vi "FY6900.vi"(4 "Error In":errorcluster, 7 "Command":T13) -> (0 "Error Out":errorcluster, 3 "Response":T11)   [LabVIEW 2018]
uses:
  MOKO_LabViewLibrary/MokoLowLevel/MokoLowLovelControl/MLLC_Command.ctl
  MOKO_LabViewLibrary/MokoLowLevel/MokoLowLovelControl/MLLC_Mode.ctl
  MOKO_LabViewLibrary/MokoLowLevel/MokoLowLovelControl/MLLC_Response.ctl
  MOKO_LabViewLibrary/MokoLowLevel/MokoLowLovelControl/MLLC_ConnectCluster.ctl
  MOKO_LabViewLibrary/MokoLowLevel/MokoLowLovelControl/MLLC_InterfaceType.ctl
  MOKO_LabViewLibrary/MokoLowLevel/MokoLowLovelControl/MLLC_OpenedSession.ctl
  MOKO_LabViewLibrary/MokoLowLevel/MokoLowLovelControl/MLLC_InterfaceSettings.ctl
  MOKO_LabViewLibrary/MokoLowLevel/MokoLowLovelControl/MLLC_InterfaceKind.ctl
  MOKO_LabViewLibrary/MokoLowLevel/MokoLowLovelControl/MLLC_DriverName.ctl
  MOKO_LabViewLibrary/MokoLowLevel/MokoLowLovelControl/MLLC_ResponseInit.ctl
  MOKO_LabViewLibrary/MokoLowLevel/MokoLowLovelControl/MLLC_Request.ctl
  MOKO_LabViewLibrary/MokoLowLevel/MokoLowLovelControl/MLLC_ErrorCode.ctl
  MOKO_LabViewLibrary/MokoLowLevel/MokoLowLovelControl/MLLC_Rs232Settings.ctl
panel:
  in  "Error Code":T1=5420
  in  "Request":T2="UMO"
  in  "ResponseInit":T3="FY6900"
  in  "Driver Name":T4="FY6900"
  in  "Settings":T10={"Saved Data"=variant, "Permanent data"={"Connect"={"InterfaceType"=enum."VISA", "OpenedSession"="", "InterfaceSettings"={"Interface"=enum."RS232", "EOS 4 read"=enum."LF (\\n)", "EOS 4 write"=enum."LF (\\n)", "TMO, ms"=2000, "Sett"=variant(cluster{"Baud Rate":u32, "Data Bits":u16, "Parity":u16, "Stop Bits":u16, "Flow Control":u16, "Eho":bool} {"Baud Rate"=75, "Data Bits"=0, "Parity"=0, "Stop Bits"=0, "Flow Control"=0, "Eho"=FALSE})}}}}
  in  "Mode":T12=enum."Check"
  # "FY6900"
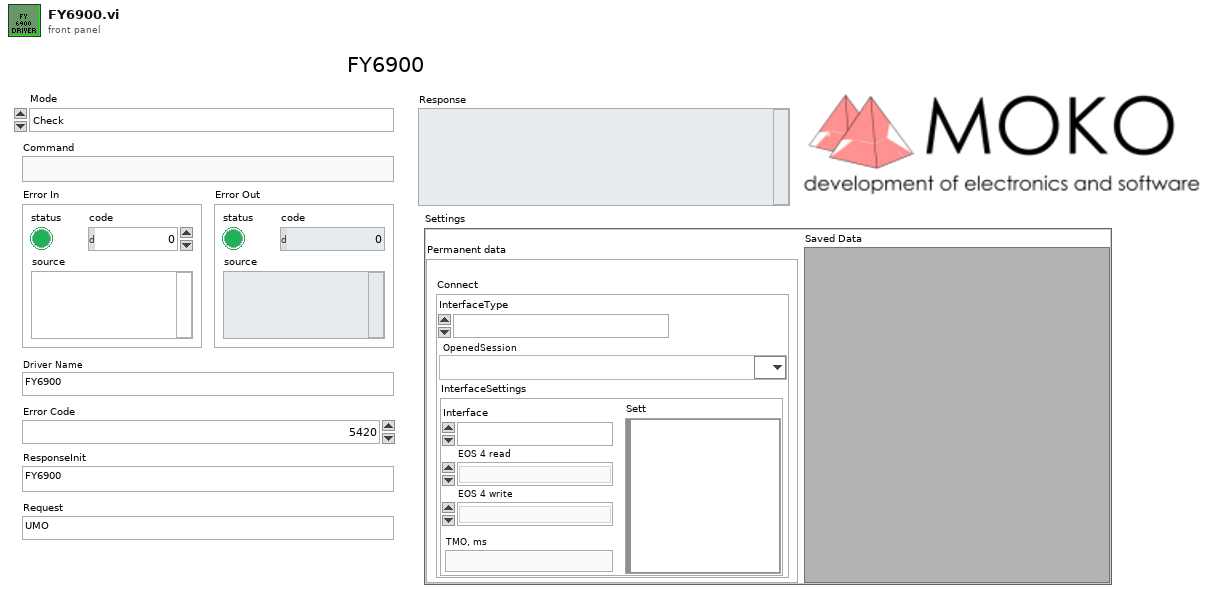
[diagram p1: front panel]
types:
  T1 = typedef "MLLC_ErrorCode.ctl" = u32
  T2 = typedef "MLLC_Request.ctl" = string
  T3 = typedef "MLLC_ResponseInit.ctl" = string
  T4 = typedef "MLLC_DriverName.ctl" = string
  T5 = typedef "MLLC_ConnectCluster.ctl" = cluster{"InterfaceType":T6, "OpenedSession":T7, "InterfaceSettings":T8}
  T6 = typedef "MLLC_InterfaceType.ctl" = enum16{"VISA", "Prologix USB-GPIB"}
  T7 = typedef "MLLC_OpenedSession.ctl" = refnum<visa-resource-name>
  T8 = typedef "MLLC_InterfaceSettings.ctl" = cluster{"Interface":T9, "EOS 4 read":enum16{"Default (=EOS 4 write)", "CR (\\r)", "LF (\\n)", "None"}, "EOS 4 write":enum16{"CR+LF (\\r\\n)", "CR (\\r)", "LF (\\n)", "None"}, "TMO, ms":i32, "Sett":variant}
  T9 = typedef "MLLC_InterfaceKind.ctl" = enum16{"RS232", "GPIB", "USB", "Ethernet", "another"}
  T10 = cluster{"Saved Data":variant, "Permanent data":cluster{"Connect":T5}}
  T11 = typedef "MLLC_Response.ctl" = string
  T12 = typedef "MLLC_Mode.ctl" = enum16{"get", "set", "close", "Init", "Check"}
  T13 = typedef "MLLC_Command.ctl" = string
  T14 = enum16{"CR+LF (\\r\\n)", "CR (\\r)", "LF (\\n)", "None"}
  T15 = enum16{"Default (=EOS 4 write)", "CR (\\r)", "LF (\\n)", "None"}
  T16 = typedef "MLLC_Error.ctl" = errorcluster
  T17 = typedef "MLLC_Rs232Settings.ctl" = cluster{"Baud Rate":u32, "Data Bits":u16, "Parity":u16, "Stop Bits":u16, "Flow Control":u16, "Eho":bool}
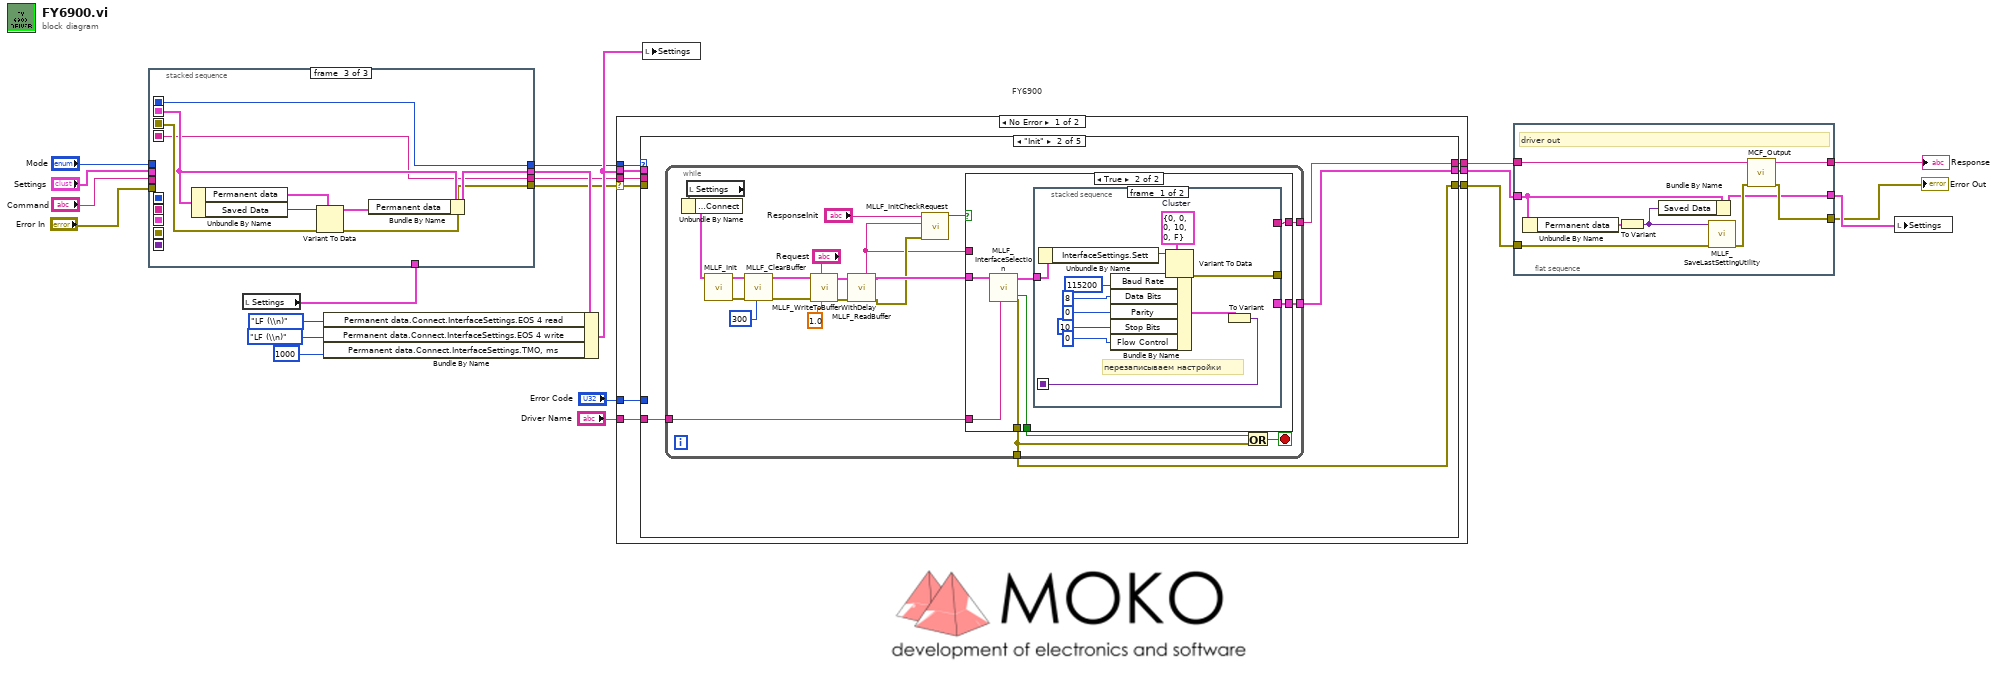
[diagram p0: block diagram]
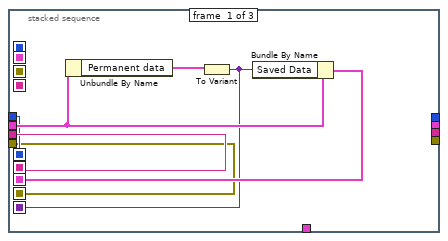
[diagram p2: hidden frame]
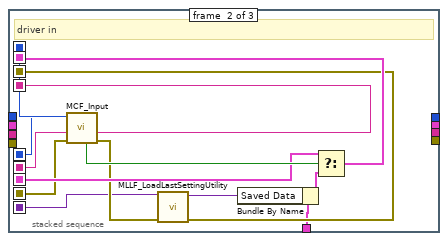
[diagram p3: hidden frame]
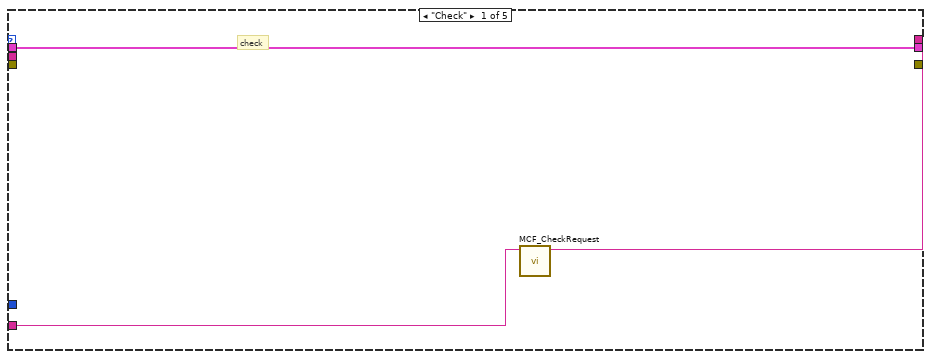
[diagram p4: hidden frame]
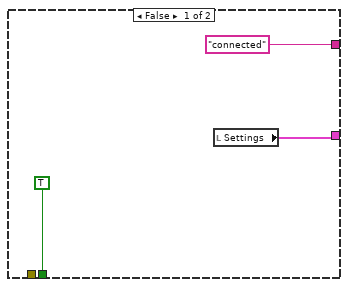
[diagram p5: hidden frame]
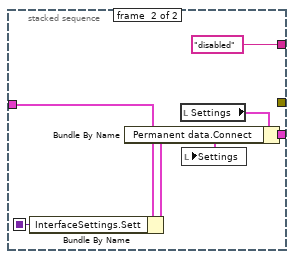
[diagram p6: hidden frame]
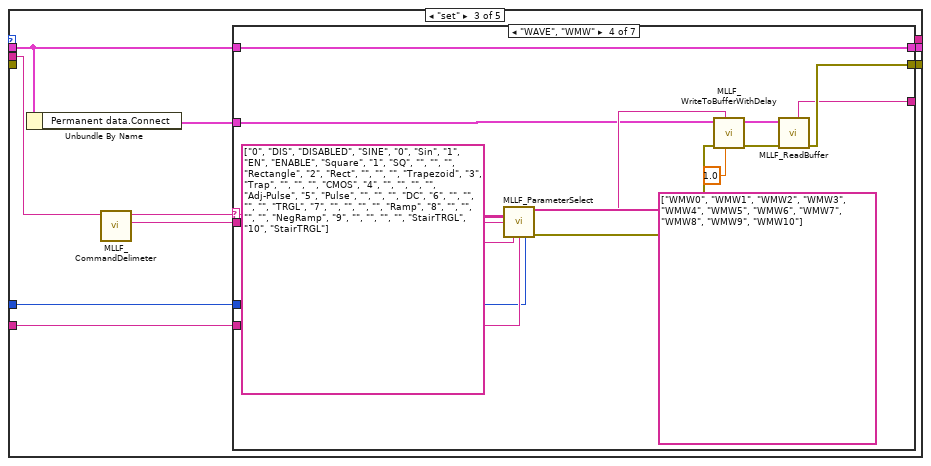
[diagram p7: hidden frame]
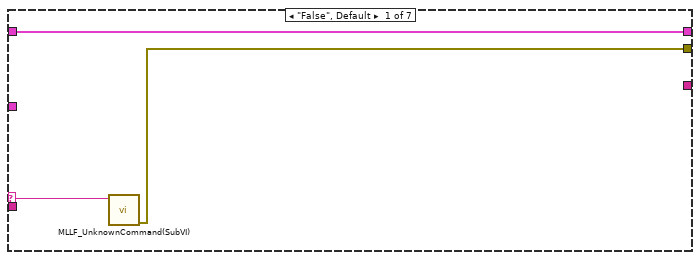
[diagram p8: hidden frame]
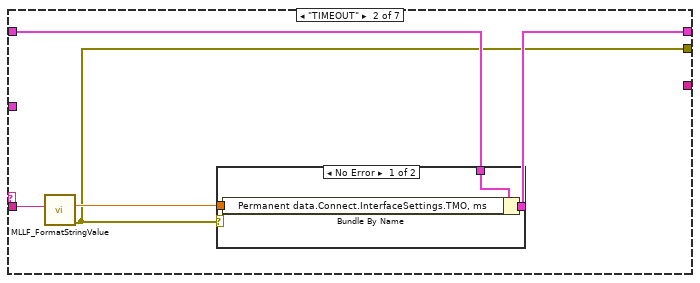
[diagram p9: hidden frame]
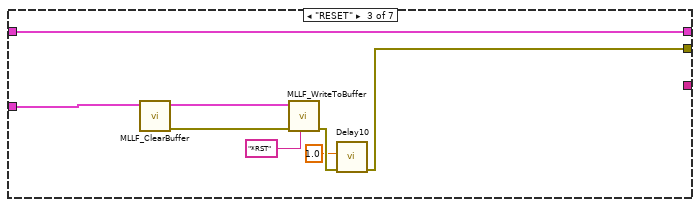
[diagram p11: hidden frame]
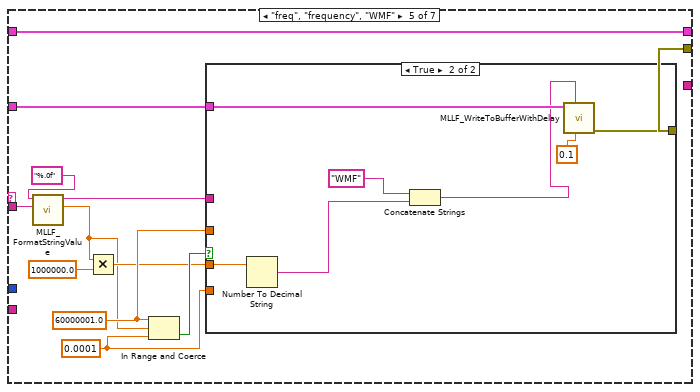
[diagram p12: hidden frame]
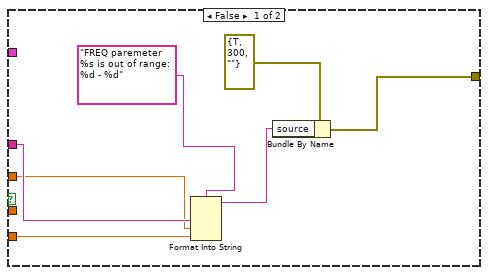
[diagram p13: hidden frame]
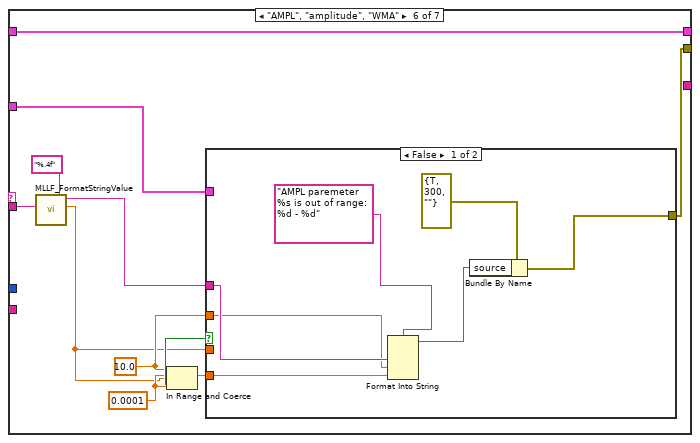
[diagram p14: hidden frame]
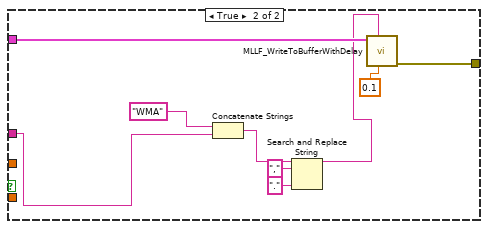
[diagram p15: hidden frame]
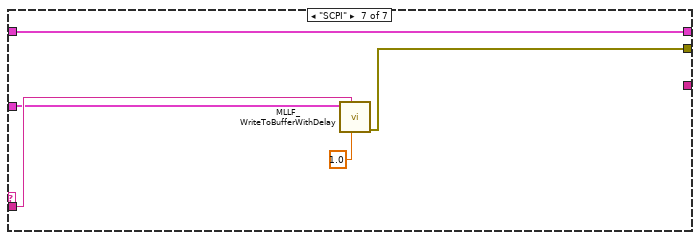
[diagram p16: hidden frame]
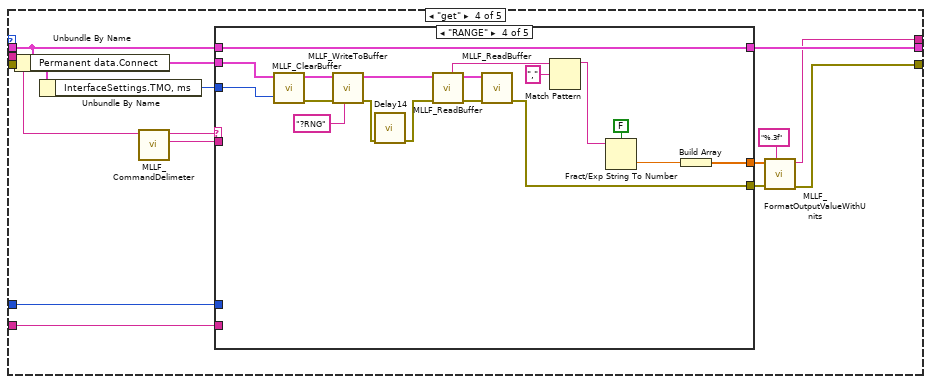
[diagram p17: hidden frame]
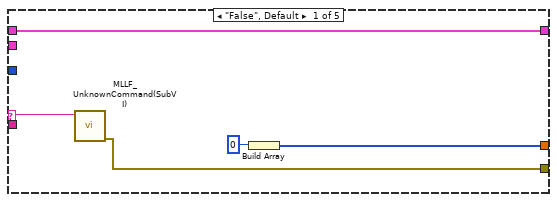
[diagram p18: hidden frame]
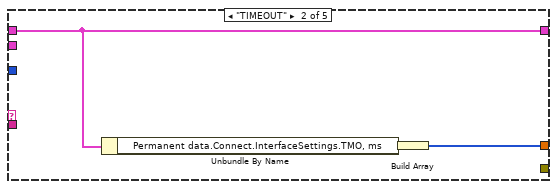
[diagram p19: hidden frame]
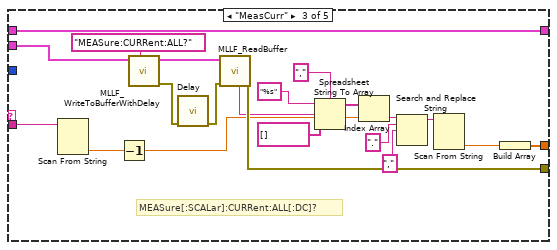
[diagram p20: hidden frame]
diagram:
  # "FY6900"
  n1 = local read "Settings"() -> (w5:T10)
  n2 = stacked-sequence {
    seq-local: [w24 _ _] -> [_ w40 _]
    seq-local: [w23 _ _] -> [_ w41 _]
    seq-local: [w26 _ _] -> [_ w36 _]
    seq-local: [w22 _ _] -> [_ w35 _]
    seq-local: [w25 _ _] -> [_ w31 _]
    seq-local: [_ w32 _] -> [_ _ w48]
    seq-local: [_ w42 _] -> [_ _ w45]
    seq-local: [_ w39 _] -> [_ _ w44]
    seq-local: [_ w38 _] -> [_ _ w49]
    tunnel: "Command" -> [w24 _ _]
    tunnel: "Mode" -> [w23 _ _]
    tunnel: "Error In" -> [w22 _ _]
    tunnel: "Settings" -> [w27 _ _]
    tunnel: w5 -> [_ w30 _]
    tunnel: [_ _ w44] -> w2
    tunnel: [_ _ w47] -> w4
    tunnel: [_ _ w46] -> w1
    tunnel: [_ _ w45] -> w3
    frame #0 {
      n3 = Unbundle By Name(w27) -> ("Permanent data"=w28:cluster{"Connect":T5})
      n4 = To Variant(anything=w28) -> (Variant=w25:variant)
      n5 = Bundle By Name(cluster=w27, "Saved Data"=w25) -> (w26:T10)
    }
    frame #1 {
      # "driver in"
      n6 = call "MCF_Input.vi"("Error In"=w35, "Command in"=w40, "Mode in"=w41) -> ("Error Out"=w34:errorcluster, "Command out"=w39:string, "Mode out"=w42:T12, "Boolean"=w37:bool)  [unwired: 5 in]
      n7 = call "MLLF_LoadLastSettingUtility.vi"("Error In"=w34, "Save data in"=w31) -> ("Error Out"=w32:errorcluster, "Save data out"=w29:variant)  [unwired: 8 in]
      n8 = Bundle By Name(cluster=w30, "Saved Data"=w29) -> (w33:T10)
      n9 = Select(t=w36, s=w37, f=w33) -> (s? t:f=w38:T10)
    }
    frame #2 {
      n10 = Unbundle By Name(w49) -> ("Permanent data"=w50:cluster{"Connect":T5}, "Saved Data"=w43:variant)
      n11 = Variant To Data(error in=w48, type=w50, Variant=w43) -> (data=w51:cluster{"Connect":T5}, error out=w46:errorcluster)
      n12 = Bundle By Name(cluster=w49, "Permanent data"=w51) -> (w47:T10)
    }
  }
  n13 = Bundle By Name(cluster=w4, "Permanent data.Connect.InterfaceSettings.EOS 4 read"=T15."LF (\\n)" ("Connect.InterfaceSettings.EOS 4 read"), "Permanent data.Connect.InterfaceSettings.EOS 4 write"=T14."LF (\\n)" ("Connect.InterfaceSettings.EOS 4 write"), "Permanent data.Connect.InterfaceSettings.TMO, ms"=1000 ("Connect.InterfaceSettings.TMO, ms")) -> (w19:T10)
  n14 = case shown="No Error" w1 {
    selector: w1 -> [w56 w303]
    tunnel: [w58 w303] -> w13
    tunnel: w3 -> [w60 _]
    tunnel: [w59 _] -> w15
    tunnel: w2 -> [w57 _]
    tunnel: w19 -> [w53 w302]
    tunnel: "Error Code" -> [w55 _]
    tunnel: "Driver Name" -> [w54 _]
    tunnel: [w52 w302] -> w14
    frame No Error {
      n15 = case shown="\"Init\"" w60 {
        tunnel: [w61 w65 _ w220 "" ("Output String")] -> w59
        tunnel: [_ w67 w121 w221 w300] -> w58
        tunnel: w57 -> [_ _ w120 w226 _]
        tunnel: w56 -> [_ _ _ _ _]
        tunnel: w55 -> [_ _ w126 w230 _]
        tunnel: w54 -> [w62 w64 w123 w229 _]
        tunnel: w53 -> [w63 _ w125 w232 w299]
        tunnel: [w63 w66 w124 w231 w299] -> w52
        frame "Check" {
          # "check"
          n16 = call "MCF_CheckRequest.vi"("Driver Name"=w62) -> ("Output String"=w61:string)  [unwired: 9 in, 1 out]
        }
        frame "Init" {
          n17 = while {
            tunnel: [w83] -> w67
            tunnel: [w80] -> w66
            tunnel: [w79] -> w65
            tunnel: w64 -> [w73]
            stop <- w85 stop-if-true
            n18 = local read "Settings"() -> (w89:T10)
            n19 = Unbundle By Name(w89) -> ("Permanent data.Connect"=w86:T5)
            n20 = call "MLLF_Init.vi"("DriverConnect in"=w86) -> ("Error Out"=w75:errorcluster, "DriverConnect out"=w76:T5)  [unwired: 7 in]
            n21 = call "MLLF_ClearBuffer.vi"("Timeout"=u32 300, "Error In"=w75, "DriverConnect in"=w76) -> ("Error Out"=w71:errorcluster, "DriverConnect out"=w72:T5)  [unwired: 5 in, 1 out]
            n22 = call "MLLF_WriteToBufferWithDelay.vi"("Delay Time ( 0,05 s)"=1.0 ("Delay Time (s)"), "Command"="Request", "Error In"=w71, "DriverConnect in"=w72) -> ("Error Out"=w82:errorcluster, "DriverConnect out"=w88:T5)  [unwired: 6 in]
            n23 = call "MLLF_ReadBuffer.vi"("Error In"=w82, "DriverConnect in"=w88) -> ("Error Out"=w69:errorcluster, "DriverConnect out"=w70:T5, "String"=w68:string)  [unwired: 6 in]
            n24 = call "MLLF_InitCheckRequest.vi"("error in (no error)"=w69, "Answer"=w68, "Response Init"="ResponseInit") -> ("Design"=w77:bool)  [unwired: 5 in, 3 out]
            n25 = case shown="True" w77 {
              tunnel: w70 -> [_ w98]
              tunnel: [TRUE w94] -> w84
              tunnel: [_ w99] -> w83
              tunnel: [w90 w96] -> w80
              tunnel: ["connected" w95] -> w79
              tunnel: w68 -> [_ _]
              tunnel: w73 -> [_ w93]
              frame False {
                n26 = local read "Settings"() -> (w90:T10)
              }
              frame True {
                n27 = call "MLLF_InterfaceSelection.vi"("Driver Name"=w93, "DriverConnect in"=w98) -> ("error out"=w99:T16, "DriverConnect out"=w97:T5, "stop init?"=w94:bool)  [unwired: 7 in]
                n28 = stacked-sequence {
                  seq-local: [w102 _] -> [_ w116]
                  tunnel: w97 -> [w101 w113]
                  tunnel: [w103 _] -> _
                  tunnel: [_ w115] -> w96
                  tunnel: [_ "disabled"] -> w95
                  frame #0 {
                    w105 = T17 {"Baud Rate"=0, "Data Bits"=0, "Parity"=0, "Stop Bits"=10, "Flow Control"=0, "Eho"=FALSE}  # Cluster
                    # "перезаписываем настройки"
                    n29 = Unbundle By Name(w101) -> ("InterfaceSettings.Sett"=w104:variant)
                    n30 = Variant To Data(type=w105, Variant=w104) -> (data=w106:T17, error out=w103:errorcluster)  [unwired: 1 in]
                    n31 = Bundle By Name(cluster=w106, "Baud Rate"=u32 115200, "Data Bits"=u16 8 ("Serial Settings:Data Bits"), "Parity"=u16 0 ("Serial Settings:Parity"), "Stop Bits"=u16 10 ("Serial Settings:Stop Bits"), "Flow Control"=u16 0 ("Serial Settings:Flow Control")) -> (w111:T17)
                    n32 = To Variant(anything=w111) -> (Variant=w102:variant)
                  }
                  frame #1 {
                    n33 = Bundle By Name(cluster=w113, "InterfaceSettings.Sett"=w116) -> (w112:T5)
                    n34 = local read "Settings"() -> (w117:T10)
                    n35 = Bundle By Name(cluster=w117, "Permanent data.Connect"=w112) -> (w115:T10)
                    n36 = local write "Settings"(w115) -> ()
                  }
                }
              }
            }
            n37 = Or(x=w84, y=w83) -> (x .or. y?=w85:bool)
          }
        }
        frame "set" {
          n38 = Unbundle By Name(w125) -> ("Permanent data.Connect"=w122:T5)
          n39 = call "MLLF_CommandDelimeter.vi"("command with param"=w120) -> ("param 1"=w118:string, "command"=w119:string)  [unwired: 6 in, 3 out]
          n40 = case shown="\"WAVE\", \"WMW\"" w119 {
            selector: w119 -> [w128 _ _ w151 _ _ _]
            tunnel: w118 -> [_ w132 _ w160 w169 w193 w216]
            tunnel: w126 -> [_ _ _ w156 _ _ _]
            tunnel: w125 -> [w129 w133 w146 w161 w162 w188 w218]
            tunnel: [w129 w134 w146 w161 w162 w188 w218] -> w124
            tunnel: w122 -> [_ _ w144 w152 w168 w189 w215]
            tunnel: w123 -> [_ _ _ w157 _ _ _]
            tunnel: [w127 w130 w139 w148 w167 w192 w214] -> w121
            tunnel: [_ _ _ w147 _ _ _] -> _
            frame "False", Default {
              n41 = call "MLLF_UnknownCommand(SubVI).vi"("Unknown command"=w128) -> ("error out"=w127:errorcluster)  [unwired: 10 in]
            }
            frame "TIMEOUT" {
              n42 = call "MLLF_FormatStringValue.vi"("String Value"=w132) -> ("error out"=w130:T16, "number"=w131:dbl)  [unwired: 8 in, 1 out]
              n43 = case shown="No Error" w130 {
                tunnel: [w137 w138] -> w134
                tunnel: w133 -> [w136 w138]
                tunnel: w131 -> [w135 _]
                frame No Error {
                  n44 = Bundle By Name(cluster=w136, "Permanent data.Connect.InterfaceSettings.TMO, ms"=w135) -> (w137:T10)
                }
                frame Error {
                }
              }
            }
            frame "RESET" {
              n45 = call "MLLF_ClearBuffer.vi"("DriverConnect in"=w144) -> ("Error Out"=w143:errorcluster, "DriverConnect out"=w142:T5)  [unwired: 7 in, 1 out]
              n46 = call "MLLF_WriteToBuffer.vi"("String"="*RST", "error in"=w143, "DriverConnect in"=w142) -> ("error out"=w141:T16)  [unwired: 5 in, 1 out]
              n47 = call "Delay10"("error in (no error)"=w141, "Delay Time (s)"=1.0) -> ("error out"=w139:errorcluster)  [unwired: 9 in]
            }
            frame "WAVE", "WMW" {
              n48 = call "MLLF_ParameterSelect.vi"("Command to equipment"=string[] ["WMW0", "WMW1", "WMW2", "WMW3", "WMW4", "WMW5", "WMW6", "WMW7", "WMW8", "WMW9", "WMW10"] ("Names"), "Names"=string[][] [["0", "DIS", "DISABLED", "SINE", "0", "Sin"], ["1", "EN", "ENABLE", "Square", "1", "SQ"], ["", "", "", "Rectangle", "2", "Rect"], ["", "", "", "Trapezoid", "3", "Trap"], ["", "", "", "CMOS", "4", ""], ["", "", "", "Adj-Pulse", "5", "Pulse"], ["", "", "", "DC", "6", ""], ["", "", "", "TRGL", "7", ""], ["", "", "", "Ramp", "8", ""], ["", "", "", "NegRamp", "9", ""], ["", "", "", "StairTRGL", "10", "StairTRGL"]], "Input"=w160, "Command"=w151, "Driver Name"=w157, "Error Code"=w156) -> ("Choice"=w153:string, "Error Out"=w154:errorcluster)  [unwired: 8 in]
              n49 = call "MLLF_WriteToBufferWithDelay.vi"("Delay Time ( 0,05 s)"=1.0 ("Delay Time (s)"), "Command"=w153, "Error In"=w154, "DriverConnect in"=w152) -> ("Error Out"=w150:errorcluster, "DriverConnect out"=w149:T5)  [unwired: 6 in]
              n50 = call "MLLF_ReadBuffer.vi"("Error In"=w150, "DriverConnect in"=w149) -> ("Error Out"=w148:errorcluster, "String"=w147:string)  [unwired: 6 in, 1 out]
            }
            frame "freq", "frequency", "WMF" {
              w171 = 0.0001 ("lower limit")
              w170 = 60000001.0 ("upper limit")
              n51 = call "MLLF_FormatStringValue.vi"("String Value"=w169, "Format"=T13 "%.0f") -> ("number"=w163:dbl, "String Value Formated"=w172:T13)  [unwired: 7 in, 1 out]
              n52 = Multiply(x=w163, y=1000000.0) -> (x*y=w164:dbl)
              n53 = In Range and Coerce(upper limit=w170, x=w163, lower limit=w171) -> (In Range?=w173:bool)  [unwired: 1 out]
              n54 = case shown="True" w173 {
                tunnel: w168 -> [_ w186]
                tunnel: [w179 w183] -> w167
                tunnel: w172 -> [w178 _]
                tunnel: w171 -> [w175 _]
                tunnel: w170 -> [w174 _]
                tunnel: w164 -> [_ w182]
                frame False {
                  n55 = Format Into String(format string="FREQ paremeter %s is out of range: %d - %d", w178, w174, w175) -> (resulting string=w177:string)  [unwired: 2 in, 1 out]
                  n56 = Bundle By Name(cluster=errorcluster {"status"=TRUE, "code"=300, "source"=""} ("Error Out"), "source"=w177) -> (w179:errorcluster)
                }
                frame True {
                  n57 = Number To Decimal String(number=w182) -> (decimal integer string=w181:string)  [unwired: 1 in]
                  n58 = Concatenate Strings(T13 "WMF" ("Command"), w181) -> (w185:string)
                  n59 = call "MLLF_WriteToBufferWithDelay.vi"("Delay Time ( 0,05 s)"=0.1 ("Delay Time (s)"), "Command"=w185, "DriverConnect in"=w186) -> ("Error Out"=w183:errorcluster)  [unwired: 7 in, 1 out]
                }
              }
            }
            frame "AMPL", "amplitude", "WMA" {
              w195 = 0.0001 ("lower limit")
              w194 = 10.0 ("upper limit")
              n60 = call "MLLF_FormatStringValue.vi"("String Value"=w193, "Format"=T13 "%.4f") -> ("number"=w190:dbl, "String Value Formated"=w196:T13)  [unwired: 7 in, 1 out]
              n61 = In Range and Coerce(upper limit=w194, x=w190, lower limit=w195) -> (In Range?=w197:bool)  [unwired: 1 out]
              n62 = case shown="False" w197 {
                tunnel: w189 -> [_ w212]
                tunnel: [w203 w210] -> w192
                tunnel: w196 -> [w202 w209]
                tunnel: w195 -> [w199 _]
                tunnel: w194 -> [w198 _]
                tunnel: w190 -> [_ _]
                frame False {
                  n63 = Format Into String(format string="AMPL paremeter %s is out of range: %d - %d", w202, w198, w199) -> (resulting string=w201:string)  [unwired: 2 in, 1 out]
                  n64 = Bundle By Name(cluster=errorcluster {"status"=TRUE, "code"=300, "source"=""} ("Error Out"), "source"=w201) -> (w203:errorcluster)
                }
                frame True {
                  n65 = Concatenate Strings(T13 "WMA" ("Command"), w209) -> (w208:string)
                  n66 = Search and Replace String(input string=w208, search string=",", replace string="." ("replace string (\"\")")) -> (result string=w205:string)  [unwired: 5 in, 3 out]
                  n67 = call "MLLF_WriteToBufferWithDelay.vi"("Delay Time ( 0,05 s)"=0.1 ("Delay Time (s)"), "Command"=w205, "DriverConnect in"=w212) -> ("Error Out"=w210:errorcluster)  [unwired: 7 in, 1 out]
                }
              }
            }
            frame "SCPI" {
              n68 = call "MLLF_WriteToBufferWithDelay.vi"("Delay Time ( 0,05 s)"=1.0 ("Delay Time (s)"), "Command"=w216, "DriverConnect in"=w215) -> ("Error Out"=w214:errorcluster)  [unwired: 7 in, 1 out]
            }
          }
        }
        frame "get" {
          n69 = Unbundle By Name(w232) -> ("Permanent data.Connect"=w223:T5)
          n70 = Unbundle By Name(w223) -> ("InterfaceSettings.TMO, ms"=w222:i32)
          n71 = call "MLLF_CommandDelimeter.vi"("command with param"=w226) -> ("param 1"=w224:string, "command"=w225:string)  [unwired: 6 in, 3 out]
          n72 = case shown="\"RANGE\"" w225 {
            selector: w225 -> [w234 _ _ _ _]
            tunnel: w224 -> [_ _ w251 _ _]
            tunnel: [w233 _ w256 w270 w288] -> w228
            tunnel: w230 -> [_ _ _ _ _]
            tunnel: [w237 w240 w261 w279 w297] -> w231
            tunnel: w232 -> [w237 w240 w261 w279 w297]
            tunnel: [w235 w238 w260 w276 w294] -> w227
            tunnel: w223 -> [_ _ w241 w274 w292]
            tunnel: w229 -> [_ _ _ _ _]
            tunnel: w222 -> [_ _ _ w273 w291]
            frame "False", Default {
              n73 = call "MLLF_UnknownCommand(SubVI).vi"("Unknown command"=w234) -> ("error out"=w233:errorcluster)  [unwired: 10 in]
              n74 = Build Array(0 ("TimeOut")) -> (w235:i32[])
            }
            frame "TIMEOUT" {
              n75 = Unbundle By Name(w240) -> ("Permanent data.Connect.InterfaceSettings.TMO, ms"=w239:i32)
              n76 = Build Array(w239) -> (w238:i32[])
            }
            frame "MeasCurr" {
              # "MEASure[:SCALar]:CURRent:ALL[:DC]?"
              n77 = Scan From String(input string=w251) -> (output 1=w246:dbl)  [unwired: 4 in, 3 out]
              n78 = Decrement(x=w246) -> (x-1=w245:dbl)
              n79 = call "MLLF_WriteToBufferWithDelay.vi"("Command"="MEASure:CURRent:ALL?" ("String"), "DriverConnect in"=w241) -> ("Error Out"=w258:errorcluster, "DriverConnect out"=w242:T5)  [unwired: 8 in]
              n80 = call "Delay"("error in (no error)"=w258) -> ("error out"=w257:errorcluster)  [unwired: 10 in]
              n81 = call "MLLF_ReadBuffer.vi"("Error In"=w257, "DriverConnect in"=w242) -> ("Error Out"=w256:errorcluster, "String"=w250:string)  [unwired: 6 in, 1 out]
              n82 = Spreadsheet String To Array(delimiter (Tab)=",", format string="%s", spreadsheet string=w250, array type (2D Dbl)=string[] [] ("appended array")) -> (array=w255:string[])
              n83 = Index Array(array=w255, index=w245) -> (element=w249:string)
              n84 = Search and Replace String(input string=w249, search string=".", replace string="," ("replace string (\"\")")) -> (result string=w244:string)  [unwired: 5 in, 3 out]
              n85 = Scan From String(input string=w244) -> (output 1=w243:dbl)  [unwired: 4 in, 3 out]
              n86 = Build Array(w243) -> (w260:dbl[])
            }
            frame "RANGE" {
              n87 = call "MLLF_ClearBuffer.vi"("Timeout"=w273, "DriverConnect in"=w274) -> ("Error Out"=w271:errorcluster, "DriverConnect out"=w272:T5)  [unwired: 6 in, 1 out]
              n88 = call "MLLF_WriteToBuffer.vi"("String"="?RNG", "error in"=w271, "DriverConnect in"=w272) -> ("error out"=w263:T16, "DriverConnect out"=w267:T5)  [unwired: 5 in]
              n89 = call "Delay14"("error in (no error)"=w263) -> ("error out"=w262:errorcluster)  [unwired: 10 in]
              n90 = call "MLLF_ReadBuffer.vi"("Error In"=w262, "DriverConnect in"=w267) -> ("Error Out"=w266:errorcluster, "DriverConnect out"=w265:T5, "String"=w264:string)  [unwired: 6 in]
              n91 = call "MLLF_ReadBuffer.vi"("Error In"=w266, "DriverConnect in"=w265) -> ("Error Out"=w270:errorcluster)  [unwired: 6 in, 2 out]
              n92 = Match Pattern(string=w264, regular expression=",") -> (before substring=w268:string)  [unwired: 1 in, 3 out]
              n93 = Fract/Exp String To Number(use system decimal point (T)=FALSE, string=w268) -> (number=w277:dbl)  [unwired: 2 in, 1 out]
              n94 = Build Array(w277) -> (w276:dbl[])
            }
            frame "ZERO" {
              n95 = call "MLLF_ClearBuffer.vi"("Timeout"=w291, "DriverConnect in"=w292) -> ("Error Out"=w289:errorcluster, "DriverConnect out"=w290:T5)  [unwired: 6 in, 1 out]
              n96 = call "MLLF_WriteToBuffer.vi"("String"="?Z,U", "error in"=w289, "DriverConnect in"=w290) -> ("error out"=w281:T16, "DriverConnect out"=w285:T5)  [unwired: 5 in]
              n97 = call "Delay15"("error in (no error)"=w281) -> ("error out"=w280:errorcluster)  [unwired: 10 in]
              n98 = call "MLLF_ReadBuffer.vi"("Error In"=w280, "DriverConnect in"=w285) -> ("Error Out"=w284:errorcluster, "DriverConnect out"=w283:T5, "String"=w282:string)  [unwired: 6 in]
              n99 = call "MLLF_ReadBuffer.vi"("Error In"=w284, "DriverConnect in"=w283) -> ("Error Out"=w288:errorcluster)  [unwired: 6 in, 2 out]
              n100 = Match Pattern(string=w282, regular expression=",") -> (before substring=w286:string)  [unwired: 1 in, 3 out]
              n101 = Fract/Exp String To Number(use system decimal point (T)=FALSE, string=w286) -> (number=w295:dbl)  [unwired: 2 in, 1 out]
              n102 = Build Array(w295) -> (w294:dbl[])
            }
          }
          n103 = call "MLLF_FormatOutputValueWithUnits.vi"("Format"=T13 "%.3f", "error in"=w228, "ValuesIn"=w227) -> ("error out"=w221:T16, "Result string"=w220:T13)  [unwired: 7 in]
        }
        frame "close" {
          n104 = Unbundle By Name(w299) -> ("Permanent data.Connect.OpenedSession"=w301:T7)
          n105 = VISA Close(VISA resource name=w301) -> (error out=w300:errorcluster)  [unwired: 1 in]
        }
      }
    }
    frame Error {
    }
  }
  n106 = local write "Settings"(w19) -> ()
  n107 = flat-sequence {
    tunnel: [w312] -> w12
    tunnel: [w311] -> w10
    tunnel: w15 -> [w310]
    tunnel: w13 -> [w309]
    tunnel: w14 -> [w305]
    tunnel: [w307] -> w11
    frame #0 {
      # "driver out"
      n108 = Unbundle By Name(w305) -> ("Permanent data"=w304:cluster{"Connect":T5})
      n109 = To Variant(anything=w304) -> (Variant=w306:variant)
      n110 = Bundle By Name(cluster=w305, "Saved Data"=w306) -> (w307:T10)
      n111 = call "MLLF_SaveLastSettingUtility.vi"("error in"=w309, "Saved Data"=w306) -> ("error out"=w308:T16)  [unwired: 8 in, 1 out]
      n112 = call "MCF_Output.vi"("Error In"=w308, "Input"=w310) -> ("Error Out"=w311:errorcluster, "Output"=w312:string)  [unwired: 8 in]
    }
  }
  n113 = local write "Settings"(w11) -> ()
  "Response" <- w12
  "Error Out" <- w10
